vi "Peristaltic Pump Serial interface.vi"() -> ()   [LabVIEW 2014]
uses:
  <vilib>/Instr/_visa.llb/VISA Configure Serial Port (Instr).vi
panel:
  out "?":dbl(knob) scale=0.0..41.67
  in  "?":bool
  in  "stop":bool
  in  "Steps/mL":dbl=2400.0
  out "String":string
  in  "Flow":dbl=50.0 min=0.5 max=50.0 step=0.01 format="%#_g mL/min"
  in  "Direction":u16(ring)
  in  "Volume to deliver":dbl min=0.0 max=1000.0 step=0.01 format="%#_g mL"
  in  "Deliver":bool
  in  "Pumpmode":u16(ring) items=["Off", "Continuous", "Volumetric"]
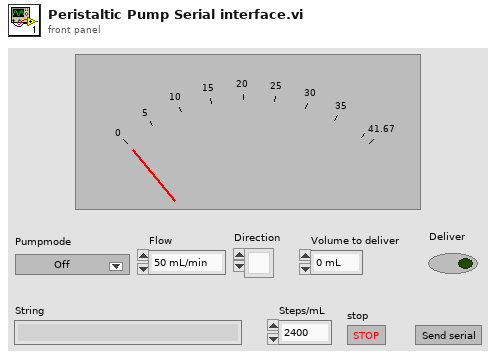
[diagram p1: front panel]
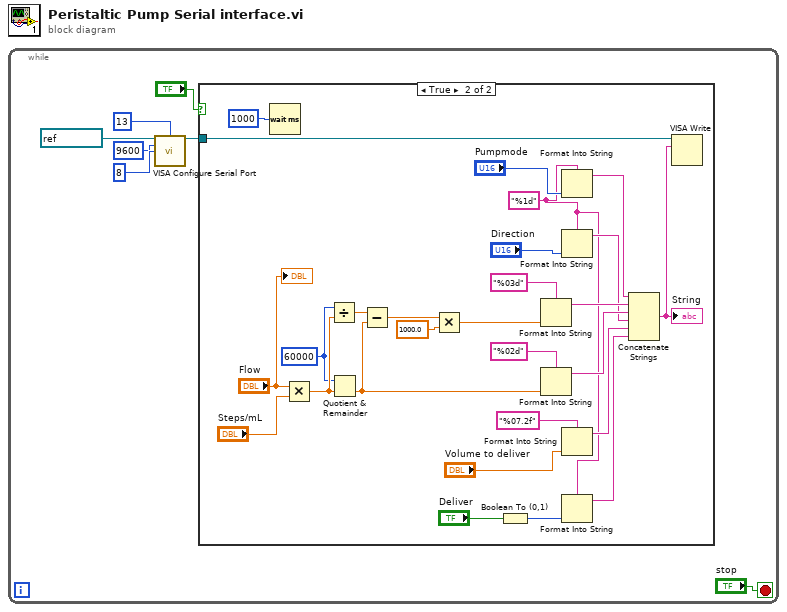
[diagram p0: block diagram]
diagram:
  n1 = while {
    stop <- "stop" stop-if-true
    n2 = call-poly "VISA Configure Serial Port"("VISA resource name"=refnum<visa-resource-name> "COM3", "termination char\n(0xA = '\\n' = LF)"=u8 13 ("termination char\n(0xA = '\\n' = LF)"), "baud rate (9600)"=u32 9600, "data bits (8)"=u16 8) -> ("VISA resource name out"=w3:refnum<visa-resource-name>)  [unwired: 10 in, 1 out]
    n3 = case shown="True" "?" {
      tunnel: w3 -> [_ w34]
      frame False {
      }
      frame True {
        w8 = 60000
        w23 = "%1d" ("format string")
        n4 = Wait (ms)(milliseconds to wait=u32 1000) -> ()  [unwired: 1 out]
        n5 = Multiply(x="Flow", y="Steps/mL") -> (x*y=w14:dbl)
        n6 = Divide(x=w8, y=w14) -> (x/y=w12:dbl)
        n7 = Quotient & Remainder(x=w8, y=w14) -> (floor(x/y)=w13:dbl)  [unwired: 1 out]
        n8 = Subtract(x=w12, y=w13) -> (x-y=w11:dbl)
        n9 = Multiply(x=w11, y=1000.0) -> (x*y=w10:dbl)
        n10 = Boolean To (0,1)(Boolean="Deliver") -> (0, 1=w25:i16)
        n11 = Format Into String(format string="%03d", w10) -> (resulting string=w30:string)  [unwired: 2 in, 1 out]
        n12 = Format Into String(format string="%02d", w13) -> (resulting string=w29:string)  [unwired: 2 in, 1 out]
        n13 = Format Into String(format string=w23, "Pumpmode") -> (resulting string=w31:string)  [unwired: 2 in, 1 out]
        n14 = Format Into String(format string=w23, "Direction") -> (resulting string=w28:string)  [unwired: 2 in, 1 out]
        n15 = Format Into String(format string="%07.2f", "Volume to deliver") -> (resulting string=w27:string)  [unwired: 2 in, 1 out]
        n16 = Format Into String(format string=w23, w25) -> (resulting string=w26:string)  [unwired: 2 in, 1 out]
        n17 = Concatenate Strings(w31, w30, w29, w28, w27, w26) -> (w19:string)
        "String" <- w19
        n18 = VISA Write(VISA resource name=w34, write buffer=w19) -> ()  [unwired: 1 in, 3 out]
        "?" <- "Flow"
      }
    }
  }
